vi "Initialize Subpanel to Main Command.vi"(8 "error in (no error)":errorcluster) -> (0 "error out":errorcluster, 2 "subpanel to main command event reg":T2, 3 "subpanel to main command event":T1)   [LabVIEW 2017, in "NI_Robotics_Configure Steering Frame.lvlib"]
uses:
  <vilib>/robotics/Dialog/Configure Steering Frame/NI_Robotics_Configure Steering Frame.lvlib
  <vilib>/robotics/Dialog/Configure Steering Frame/Subpanel to Main Command Event Reg.ctl
  <vilib>/robotics/Dialog/Configure Steering Frame/Subpanel to Main Command Event.ctl
  <vilib>/robotics/Dialog/Configure Steering Frame/Subpanel to Main Command.ctl
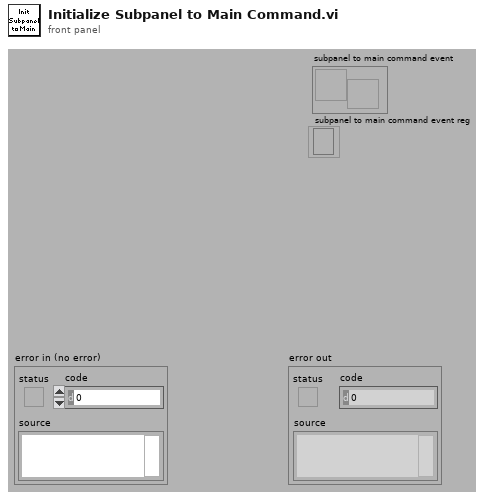
[diagram p1: front panel]
types:
  T1 = typedef "NI_Robotics_Configure Steering Frame.lvlib/Subpanel to Main Command Event.ctl" = refnum<user-event>
  T2 = typedef "NI_Robotics_Configure Steering Frame.lvlib/Subpanel to Main Command Event Reg.ctl" = refnum<event-registration>
  T3 = typedef "NI_Robotics_Configure Steering Frame.lvlib/Subpanel to Main Command.ctl" = cluster{"command":string, "data":variant}
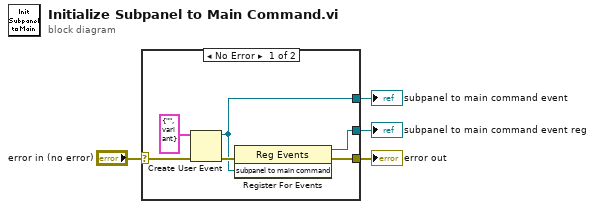
[diagram p0: block diagram]
diagram:
  n1 = case shown="No Error" "error in (no error)" {
    selector: "error in (no error)" -> [w9 w11]
    tunnel: [w7 _] -> w3
    tunnel: [w6 _] -> w1
    tunnel: [w5 w11] -> w2
    frame No Error {
      n2 = Create User Event(user event datatype=T3 {"command"="", "data"=variant} ("subpanel to main command"), error in=w9) -> (user event=w7:refnum<user-event>, error out=w8:errorcluster)
      n3 = register-events(error in=w8, w7) -> (reference out=w6:refnum<event-registration>, error out=w5:errorcluster)  [unwired: 1 in]
    }
    frame Error {
    }
  }
  "error out" <- w2
  "subpanel to main command event reg" <- w1
  "subpanel to main command event" <- w3
